vi "DO N Samples.vi"() -> ()   [LabVIEW 2019]
uses:
  <vilib>/Platform/TimedLoop/XDataNode/timing_clust.ctl
  <vilib>/Platform/TimedLoop/XDataNode/nitl_modes.ctl
  <vilib>/Platform/TimedLoop/XDataNode/wakeup.ctl
  <vilib>/rvi/Emulation/niFpgaSctlEmulationGetInTimedLoop.vi
  <vilib>/rvi/Emulation/niFpgaEmulationReportErrorSimple.vi
  <vilib>/rvi/Emulation/niFpgaGetClockAttributes.vi
  <vilib>/rvi/Emulation/niFpgaCriticalErrorInLSC.vi
  <vilib>/Platform/TimedLoop/XDataNode/XDataNode.xnode
  <vilib>/Platform/TimedLoop/XDataNode/XDNodeRunTimeDep.lvlib
panel:
  in  "DO.A.DMA_ENA":fxp<+,20,20> format="%020b"
  out "DO.A.DMA_IDL":bool
  in  "DO.A.DMA_CNTR":u16 format="%.0b"
  in  "DIO.A_19:0.OUT":fxp<+,20,20> format="%.0b"
  out "DIO.A_19:0.IN":fxp<+,20,20> format="%.0b"
  in  "DIO.A_19:0.DIR":fxp<+,20,20> format="%.0b"
  in  "DO.B.DMA_CNTR":u16 format="%.0b"
  out "DO.B.DMA_IDL":bool
  in  "DO.B.DMA_ENA":fxp<+,20,20> format="%020b"
  in  "DIO.B_19:0.DIR":fxp<+,20,20> format="%.0b"
  out "DIO.B_19:0.IN":fxp<+,20,20> format="%.0b"
  in  "DIO.B_19:0.OUT":fxp<+,20,20> format="%.0b"
  # "Digital I/O"
  # "Digital I/O"
  # "Block Write DO"
  # "Block Write DO"
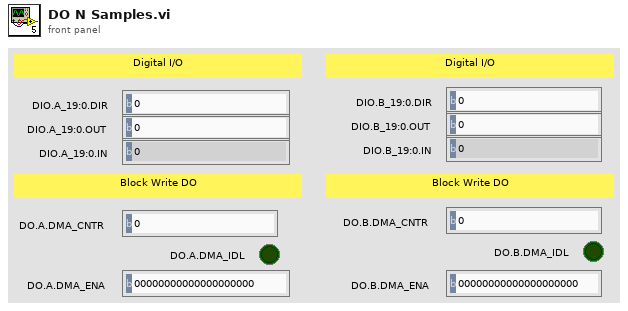
[diagram p1: front panel]
types:
  T1 = typedef "XDNodeRunTimeDep.lvlib/timing_clust.ctl" = cluster{"Expected End [f-1]":u64, "Actual End [f-1]":u64, "Finished Late? [f-1]":bool, "Expected End [i-1]":u64, "Actual End [i-1]":u64, "Finished Late? [i-1]":bool, "Expected Start [i]":u64, "Actual Start [i]":u64, "Expected Start [f]":u64, "Actual Start [f]":u64, "Source Name":string, "Structure Name":string, "Period":i64, "Deadline":i64, "Offset":i64, "Start":i64, "Priority":i32, "Timeout":i32, "Mode":T2, "Wakeup Reason":T3, "Error":errorcluster, "Source Type":string, "Secondary Source Type":string, "Global End Time":u64, "Global Start Time":u64, "Frame Duration":u64, "Iteration Duration":u64, "Assigned CPU":i32, "I/O Scan Engine Mode":u32}
  T2 = typedef "XDNodeRunTimeDep.lvlib/nitl_modes.ctl" = enum32{"No Change", "Process missed periods, maintain original phase", "Discard missed periods, maintain original phase", "Process missed periods, ignore original phase", "Discard missed periods, ignore original phase"}
  T3 = typedef "XDNodeRunTimeDep.lvlib/wakeup.ctl" = enum32{"Normal", "Aborted", "Asynchronous wakeup", "Timing source error", "Timed loop error", "Timeout"}
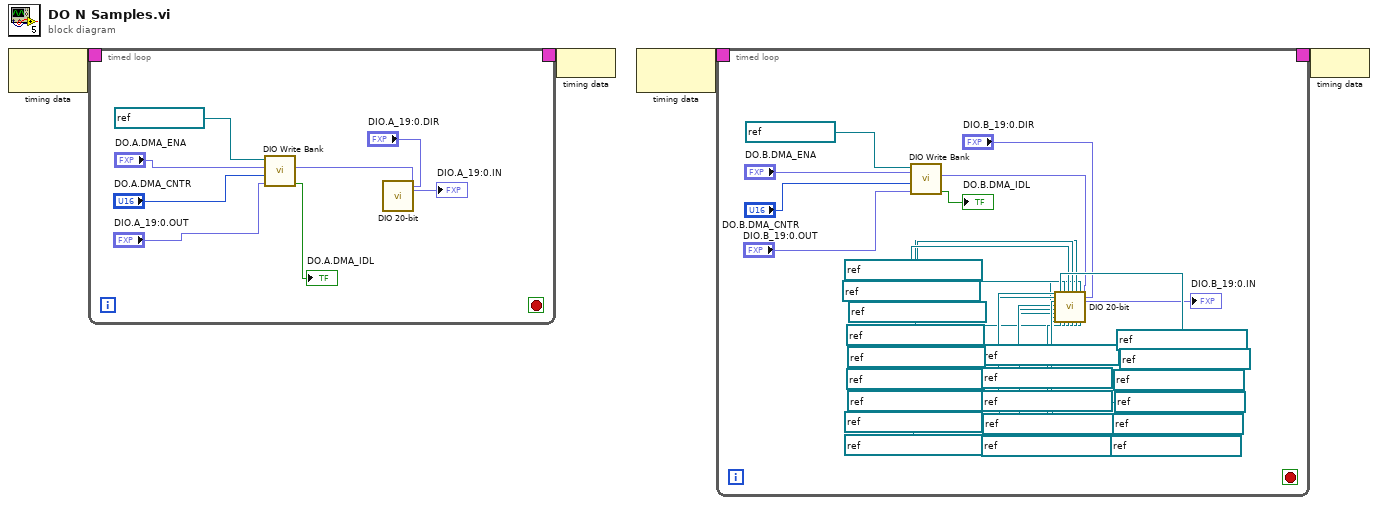
[diagram p0: block diagram]
diagram:
  n1 = node-c288() -> (w4:T1)  [unwired: 1 in]
  n2 = timed-loop {
    timing: w4 -> [_]
    timing-out: [_] -> w3
    stop <- _ stop-if-true
    n3 = call "DIO Write Bank.vi"("DIO.19:0.OUT"="DIO.A_19:0.OUT", "DO.DMA_CNTR"="DO.A.DMA_CNTR", "DO.DMA_ENA"="DO.A.DMA_ENA", "DMA FIFO IN"=refnum<k21> "DO.A.DMA") -> ("DO.DMA_IDL"=→"DO.A.DMA_IDL":bool, "DATA OUT"=w7:fxp<+,20,20>)  [unwired: 6 in]
    n4 = call "DIO 20-bit.vi"("OUT 19:0"=w7, "DIR 19:0"="DIO.A_19:0.DIR") -> ("IN 19:0"=→"DIO.A_19:0.IN":fxp<+,20,20>)  [unwired: 25 in]
  }
  n5 = node-c288(w3) -> ()
  n6 = node-c288() -> (w2:T1)  [unwired: 1 in]
  n7 = timed-loop {
    timing: w2 -> [_]
    timing-out: [_] -> w1
    stop <- _ stop-if-true
    n8 = call "DIO Write Bank.vi"("DIO.19:0.OUT"="DIO.B_19:0.OUT", "DO.DMA_CNTR"="DO.B.DMA_CNTR", "DO.DMA_ENA"="DO.B.DMA_ENA", "DMA FIFO IN"=refnum<k21> "DO.B.DMA") -> ("DO.DMA_IDL"=→"DO.B.DMA_IDL":bool, "DATA OUT"=w17:fxp<+,20,20>)  [unwired: 6 in]
    n9 = call "DIO 20-bit.vi"("DIO 0 Refnum"=refnum<k21> "ConnectorB/DIO0", "DIO 1 Refnum"=refnum<k21> "ConnectorB/DIO1", "DIO 2 Refnum"=refnum<k21> "ConnectorB/DIO2", "DIO 3 Refnum"=refnum<k21> "ConnectorB/DIO3", "DIO 4 Refnum"=refnum<k21> "ConnectorB/DIO4", "DIO 5 Refnum"=refnum<k21> "ConnectorB/DIO5", "DIO 6 Refnum"=refnum<k21> "ConnectorB/DIO6", "DIO 7 Refnum"=refnum<k21> "ConnectorB/DIO7", "DIO 8 Refnum"=refnum<k21> "ConnectorB/DIO8", "DIO 9 Refnum"=refnum<k21> "ConnectorB/DIO8", "DIO 10 Refnum"=refnum<k21> "ConnectorB/DIO10", "DIO 11 Refnum"=refnum<k21> "ConnectorB/DIO11", "DIO 12 Refnum"=refnum<k21> "ConnectorB/DIO12", "DIO 13 Refnum"=refnum<k21> "ConnectorB/DIO13", "DIO 14 Refnum"=refnum<k21> "ConnectorB/DIO16", "DIO 15 Refnum"=refnum<k21> "ConnectorB/DIO15", "DIO 16 Refnum"=refnum<k21> "ConnectorB/DIO16", "DIO 17 Refnum"=refnum<k21> "ConnectorB/DIO17", "DIO 18 Refnum"=refnum<k21> "ConnectorB/DIO18", "DIO 19 Refnum"=refnum<k21> "ConnectorB/DIO19", "OUT 19:0"=w17, "DIR 19:0"="DIO.B_19:0.DIR") -> ("IN 19:0"=→"DIO.B_19:0.IN":fxp<+,20,20>)  [unwired: 5 in]
  }
  n10 = node-c288(w1) -> ()
